vi "extractScanMode.vi"(8 "error in (no error)":errorcluster, 11 "ILC in":refnum<class "ILC.lvclass">) -> (0 "error out":errorcluster, 3 "ILC out":refnum<class "ILC.lvclass">)   [LabVIEW 2015, in "ILCCommon.lvlib" / "ILC.lvclass"]
uses:
  <userlib>/Common/ILC/ILC/ILC.lvclass
  <userlib>/Common/ILC/ILCModelTypedefs/FinalDelimiter.ctl
  <userlib>/Common/ILC/ILC/ILC.lvclass/ILC.ctl
  <userlib>/Common/ILC/Configuration/Input Channels.ctl
  <userlib>/Common/ILC/ILCModelTypedefs/ILCModelTypedefs.lvlib
  <userlib>/Common/ILC/Configuration/ILCConfiguration.lvlib
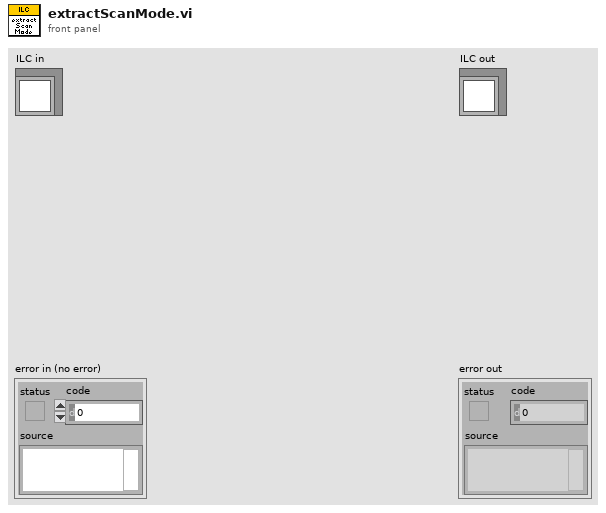
[diagram p1: front panel]
types:
  T1 = typedef "ILCCommon.lvlib/ILCModelTypedefs.lvlib/FinalDelimiter.ctl" = enum16{",", "<CR><LF>"}
  T2 = typedef "ILCCommon.lvlib/ILCConfiguration.lvlib/Input Channels.ctl" = enum16{"Channel 0", "3 Channels", "5 Channels"}
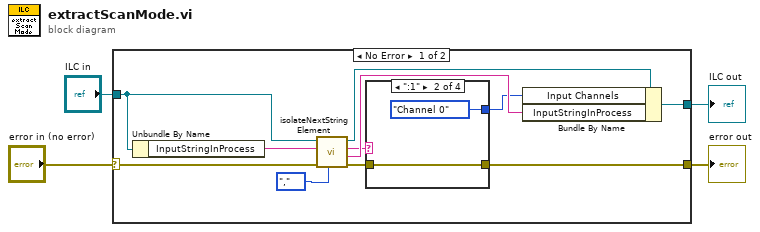
[diagram p0: block diagram]
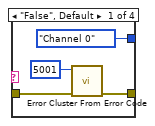
[diagram p2: hidden frame]
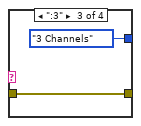
[diagram p3: hidden frame]
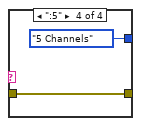
[diagram p4: hidden frame]
diagram:
  n1 = case shown="No Error" "error in (no error)" {
    selector: "error in (no error)" -> [w13 w27]
    tunnel: [w7 w27] -> w3
    tunnel: [w14 w26] -> w1
    tunnel: "ILC in" -> [w12 w26]
    frame No Error {
      n2 = Unbundle By Name(w12) -> ("InputStringInProcess"=w6:string)
      n3 = call <userlib>:"isolateNextStringElement.vi"("Final Delimiter"=FinalDelimiter.",", "error in (no error)"=w13, "inputString"=w6, "ILC in"=w12) -> ("error out"=w8:errorcluster, "remainingString"=w10:string, "extractedSegment"=w9:string, "ILC out"=w11:refnum<class "ILC.lvclass">)  [unwired: 4 in]
      n4 = case shown="\":1\"" w9 {
        tunnel: w8 -> [w18 w20 w22 w24]
        tunnel: [w17 w20 w22 w24] -> w7
        tunnel: [Input_Channels."Channel 0" ("Input Channels") Input_Channels."Channel 0" ("Input Channels") Input_Channels."3 Channels" ("Input Channels") Input_Channels."5 Channels" ("Input Channels")] -> w5
        frame "False", Default {
          n5 = call <vilib>:"Error Cluster From Error Code.vi"("error in (no error)"=w18, "error code (0)"=5001) -> ("error out"=w17:errorcluster)  [unwired: 7 in]
        }
        frame ":1" {
        }
        frame ":3" {
        }
        frame ":5" {
        }
      }
      n6 = Bundle By Name(cluster=w11, "Input Channels"=w5, "InputStringInProcess"=w10) -> (w14:refnum<class "ILC.lvclass">)
    }
    frame Error {
    }
  }
  "error out" <- w3
  "ILC out" <- w1
